vi "TablePlot.vi"(1 "表格参数":sgl[][](array[numeric]) format="%#_9g") -> (0 "Plot Pic":picture caption="通道曲线预览")   [LabVIEW 2011]
uses:
  <vilib>/picture/cartesn2.llb/XY Plot Type.ctl
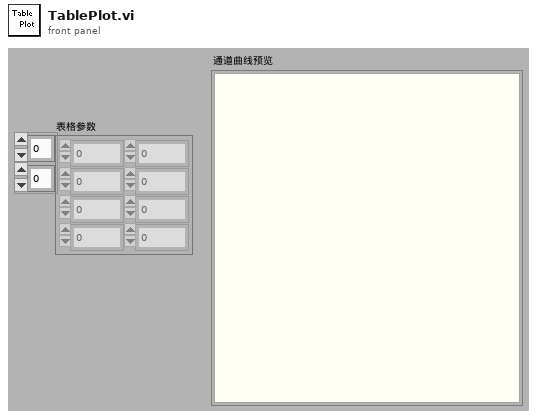
[diagram p1: front panel]
types:
  T1 = cluster{"line color":u32, "text color":u32, "tick length(3)":i16, "crossing axes":bool, "visible grid?":bool}
  T2 = typedef "XY Plot Type.ctl" = enum16{"points", "squares", "circles", "connected points", "connected squares", "connected circles", "comb plot", "sized scatter plot", "sized-colored scatter plot", "min-max lines"}
  T3 = cluster{"plot color":u32, "XY plot type":T2, "baseline":dbl}
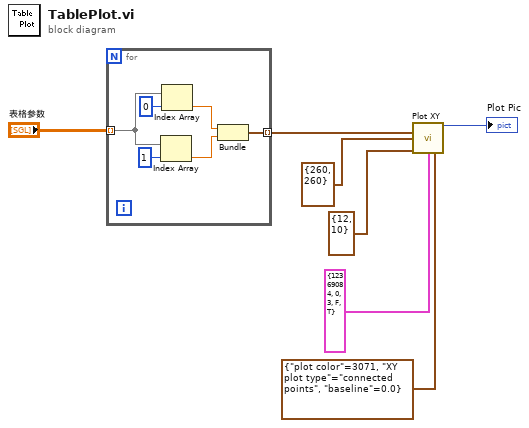
[diagram p0: block diagram]
diagram:
  n1 = for {
    tunnel: "表格参数" -> [w13] mode=indexing
    tunnel: [w8] -> w1 mode=indexing
    n2 = Index Array(array=w13, index=1) -> (element=w10:sgl)
    n3 = Index Array(array=w13, index=0) -> (element=w9:sgl)
    n4 = Bundle("Numeric"=w9, "Numeric"=w10) -> (w8:cluster{"Numeric":sgl, "Numeric":sgl})  [unwired: 1 out]
  }
  n5 = call <vilib>:"Plot XY.vi"("data"=w1, "dimensions (w,h)"=cluster{"width":i16, "height":i16} {"width"=260, "height"=260}, "top left point(0, 0)"=cluster{"x":i16, "y":i16} {"x"=12, "y"=10}, "cartesian grid cosmetics"=T1 {"line color"=12369084, "text color"=0, "tick length(3)"=3, "crossing axes"=FALSE, "visible grid?"=TRUE}, "XY plot cosmetics"=T3 {"plot color"=3071, "XY plot type"=enum."connected points", "baseline"=0.0}) -> ("new picture"=→"Plot Pic":picture)  [unwired: 2 in, 8 out]
